vi "Teleop.vi"(10 "Match Info":T1={"Autonomous Elapsed Seconds"=0.0, "TeleOp Elapsed Seconds"=0.0, "Disabled Elapsed Seconds"=0.0, "Visited Autonomous"=FALSE, "Visited TeleOp"=FALSE, "Visited Disabled"=FALSE, "Autonomous Settings"={"Autonomous Style"=enum."Independent", "VI Refnum"=refnum}}, 11 "Call Context":T2) -> ()   [LabVIEW 2016]
doc: "This VI is called for each enabled TeleOp packet received from the DS. It is typically used to read from joysticks and other inputs and update I/O or setpoints for timed control loops. It should complete and return within 20 milliseconds or risk missing DS packets."
uses:
  <vilib>/Rock Robotics/WPI/DriverStation/WPI_DriverStationDerivedRobotMode.ctl
  <vilib>/Rock Robotics/WPI/DriverStation/WPI_DriverStationMatch Info.ctl
  <vilib>/Rock Robotics/WPI/Utilities/WPI_GetSetVariantRefNum.vi
  <vilib>/Rock Robotics/Network Tables/NT Write Boolean Array.vi
  <vilib>/Rock Robotics/Network Tables/NT Write Numeric Array.vi
  Drive/Implementation/Drive Published Globals.vi
panel:
  in  "Left Setpoint":dbl=0.5 format="%#_13g"
  in  "Distance (ft)":dbl
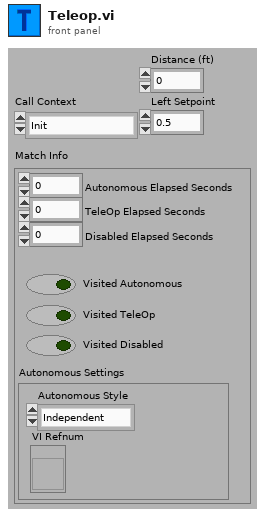
[diagram p1: front panel]
types:
  T1 = typedef "WPI_DriverStationMatch Info.ctl" = cluster{"Autonomous Elapsed Seconds":dbl, "TeleOp Elapsed Seconds":dbl, "Disabled Elapsed Seconds":dbl, "Visited Autonomous":bool, "Visited TeleOp":bool, "Visited Disabled":bool, "Autonomous Settings":cluster{"Autonomous Style":enum16{"Iterative", "Independent"}, "VI Refnum":refnum<vi>}}
  T2 = typedef "WPI_DriverStationDerivedRobotMode.ctl" = enum16{"Init", "Execute", "Stop"}
  T3 = typedef "WPI_JoystickDevRef.ctl" = cluster{"Device":T4}
  T4 = typedef "WPI_JoystickDeviceEnum.ctl" = enum16{"USB 0", "USB 1", "USB 2", "USB 3", "USB 4", "USB 5"}
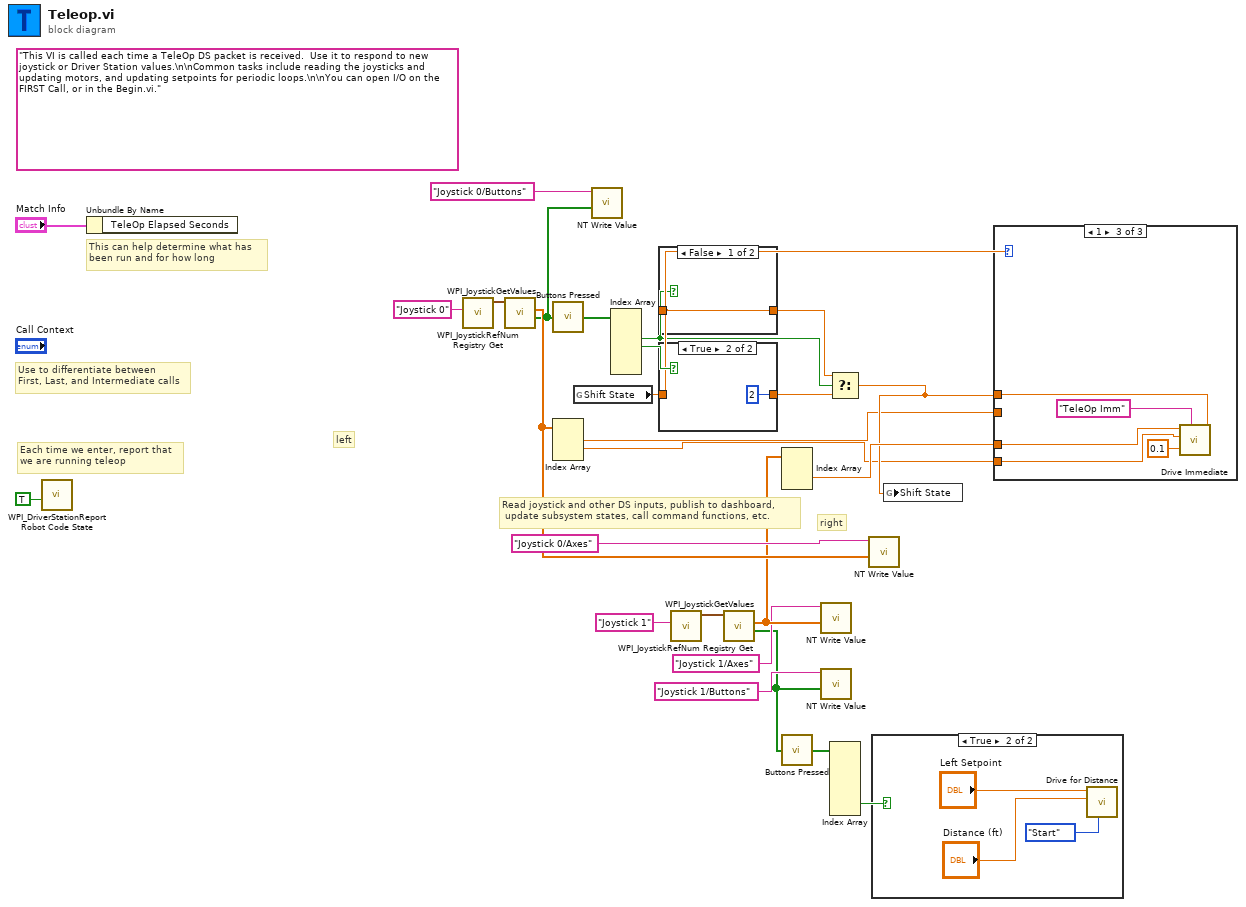
[diagram p0: block diagram]
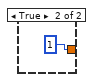
[diagram p3: hidden frame]
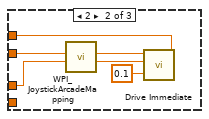
[diagram p5: hidden frame]
diagram:
  (unwired) "This VI is called each time a TeleOp DS packet is received.  Use it to respond to new joystick or Driver Station values.\n\nCommon tasks include reading the joysticks and updating motors, and updating setpoints for periodic loops.\n\nYou can open I/O on the FIRST Call, or in the Begin.vi."
  # "left"
  # "right"
  # "Read joystick and other DS inputs, publish to dashboard,\n update subsystem states, call command functions, etc."
  # "Each time we enter, report that\nwe are running teleop"
  # "Use to differentiate between\nFirst, Last, and Intermediate calls"
  # "This can help determine what has\nbeen run and for how long"
  n1 = call <vilib>:"WPI_DriverStationReport Robot Code State.vi"("TeleOp"=TRUE ("Autonomous")) -> ()  [unwired: 10 in, 1 out]
  n2 = Unbundle By Name("Match Info") -> ()  [unwired: 1 out]
  n3 = call <vilib>:"WPI_JoystickRefNum Registry Get.vi"("refnum name"="Joystick 0") -> ("JoystickDevRef"=w23:T3)  [unwired: 1 in, 9 out]
  n4 = call <vilib>:"WPI_JoystickGetValues.vi"("JoystickDevRef"=w23) -> ("Buttons"=w8:bool[], "Axes"=w21:dbl[])  [unwired: 6 in, 3 out]
  n5 = call "Buttons Pressed.vi"("Button Values"=w8) -> ("Button Presses"=w7:bool[])
  n6 = Index Array(array=w21) -> (element #1=w2:dbl, element #2=w1:dbl)  [unwired: 3 in, 1 out]
  n7 = global read "Drive Published Globals.vi" "Shift State"() -> (w9:dbl)
  n8 = call-poly <vilib>:"NT Write Value.vi"("Boolean Array"=w8, "Name"="Joystick 0/Buttons") -> ()  [unwired: 9 in, 1 out]
  n9 = Index Array(array=w7) -> (element #2=w4:bool, element #3=w10:bool)  [unwired: 6 in, 4 out]
  n10 = case shown="False" w4 {
    tunnel: [w27 1] -> w6
    tunnel: w9 -> [w27 _]
    frame False {
    }
    frame True {
    }
  }
  n11 = case shown="True" w10 {
    tunnel: [w29 2] -> w5
    tunnel: w9 -> [w29 _]
    frame False {
    }
    frame True {
    }
  }
  n12 = call <vilib>:"WPI_JoystickRefNum Registry Get.vi"("refnum name"="Joystick 1") -> ("JoystickDevRef"=w18:T3)  [unwired: 1 in, 9 out]
  n13 = call <vilib>:"WPI_JoystickGetValues.vi"("JoystickDevRef"=w18) -> ("Buttons"=w13:bool[], "Axes"=w16:dbl[])  [unwired: 6 in, 3 out]
  n14 = Index Array(array=w16) -> (element #2=w14:dbl)  [unwired: 3 in, 2 out]
  n15 = call "Buttons Pressed.vi"("Button Values"=w13) -> ("Button Presses"=w12:bool[])
  n16 = call-poly <vilib>:"NT Write Value.vi"("Numeric Array"=w16, "Name"="Joystick 1/Axes") -> ()  [unwired: 9 in, 1 out]
  n17 = call-poly <vilib>:"NT Write Value.vi"("Boolean Array"=w13, "Name"="Joystick 1/Buttons") -> ()  [unwired: 9 in, 1 out]
  n18 = Select(t=w6, s=w4, f=w5) -> (s? t:f=w3:dbl)
  n19 = Index Array(array=w12) -> (element #6=w11:bool)  [unwired: 7 in, 6 out]
  n20 = call-poly <vilib>:"NT Write Value.vi"("Numeric Array"=w21, "Name"="Joystick 0/Axes") -> ()  [unwired: 9 in, 1 out]
  n21 = case shown="True" w11 {
    frame False {
    }
    frame True {
      n22 = call "Drive for Distance.vi"("Synchronication"=enum16{"Start", "Wait"}."Start", "Distance (ft)"="Distance (ft)", "Left Setpoint"="Left Setpoint") -> ()  [unwired: 8 in, 1 out]
    }
  }
  n23 = global write "Drive Published Globals.vi" "Shift State"(w3) -> ()
  n24 = case shown="1" w9 {
    tunnel: w14 -> [_ w35 w43]
    tunnel: w3 -> [_ w36 w41]
    tunnel: w2 -> [_ w34 _]
    tunnel: w1 -> [_ _ w40]
    frame 0, Default {
    }
    frame 2 {
      n25 = call <vilib>:"WPI_JoystickArcadeMapping.vi"("Y axis value"=w35, "X axis value"=w34) -> ("Right Motor Value"=w38:dbl, "Left Motor Value"=w39:dbl)  [unwired: 8 in]
      n26 = call "Drive Immediate.vi"("Shift State"=w36, "Deadband Value"=0.1, "Right Setpoint"=w38, "Left Setpoint"=w39) -> ()  [unwired: 7 in, 1 out]
    }
    frame 1 {
      n27 = call "Drive Immediate.vi"("Shift State"=w41, "Description"="TeleOp Imm", "Deadband Value"=0.1, "Right Setpoint"=w40, "Left Setpoint"=w43) -> ()  [unwired: 6 in, 1 out]
    }
  }
